vi "Configure Sweep.vi"(5 "Frequency Stop (5E+7 Hz)":dbl=50000000.0, 6 "Frequency Step (0)":i32, 7 "Frequency Start (5E+7 Hz)":dbl=50000000.0, 8 "error in (no error)":errorcluster, 9 "Time-gated Period (0.0001 s)":dbl=0.0001, 10 "Sweep Delay (0 s)":dbl, 11 "VISA resource name":refnum<visa-resource-name>) -> (0 "error out":errorcluster, 3 "VISA resource name out":refnum<visa-resource-name>)   [LabVIEW 2018, in "Agilent U2000 Series.lvlib"]
doc: "Changes the configurations for sweep mode.\n\nNote:\nThis VI is not applicable for Agilent U2021/2XA. In case of U2040 X-Series, it's applicable for U2042XA/U2044XA/U2049XA only."
uses:
  Agilent U2000 Series.lvlib
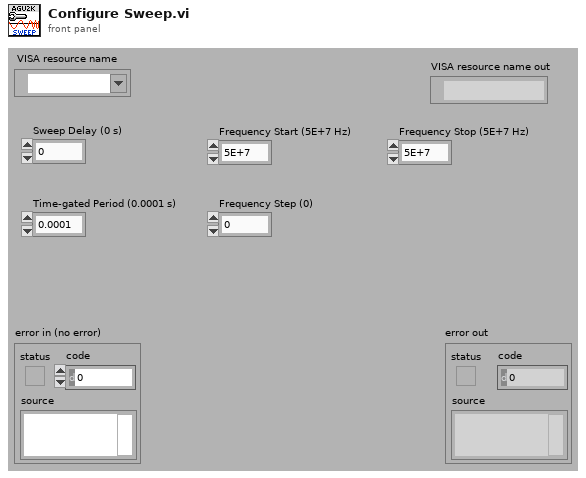
[diagram p1: front panel]
types:
  T1 = typedef "Agilent U2000 Series.lvlib/Extended User Data.ctl" = cluster{"U2000 Series Mode":u16, "Trigger Source Int/Ext":bool}
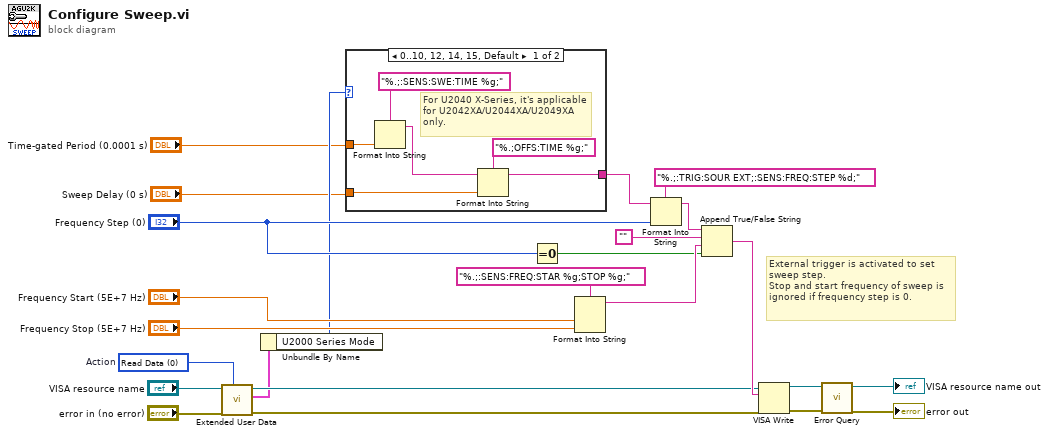
[diagram p0: block diagram]
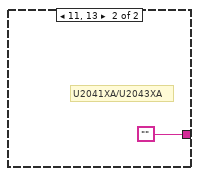
[diagram p2: hidden frame]
diagram:
  w1 = 0 items=["Read Data", "Write Data", "Clear Data", "Clear ALL Data"]  # Action
  # "External trigger is activated to set sweep step.\nStop and start frequency of sweep is ignored if frequency step is 0."
  n1 = call "Extended User Data.vi"("Action (1: Write Data)"=w1, "error in (no error)"="error in (no error)", "VISA resource name"="VISA resource name") -> ("error out"=w7:errorcluster, "User Data Out"=w6:T1, "VISA resource name out"=w8:refnum<visa-resource-name>)  [unwired: 6 in]
  n2 = Unbundle By Name(w6) -> ("U2000 Series Mode"=w5:u16)
  n3 = case shown="0..10, 12, 14, 15, Default" w5 {
    tunnel: "Time-gated Period (0.0001 s)" -> [w27 _]
    tunnel: "Sweep Delay (0 s)" -> [w26 _]
    tunnel: [w25 ""] -> w2
    frame 0..10, 12, 14, 15, Default {
      # "For U2040 X-Series, it's applicable for U2042XA/U2044XA/U2049XA only."
      n4 = Format Into String(format string="%.;:SENS:SWE:TIME %g;", w27) -> (resulting string=w28:string)  [unwired: 2 in, 1 out]
      n5 = Format Into String(format string="%.;OFFS:TIME %g;", initial string=w28, w26) -> (resulting string=w25:string)  [unwired: 1 in, 1 out]
    }
    frame 11, 13 {
      # "U2041XA/U2043XA"
    }
  }
  n6 = Equal To 0?(x="Frequency Step (0)") -> (x = 0?=w16:bool)
  n7 = Format Into String(format string="%.;:SENS:FREQ:STAR %g;STOP %g;", "Frequency Start (5E+7 Hz)", "Frequency Stop (5E+7 Hz)") -> (resulting string=w17:string)  [unwired: 2 in, 1 out]
  n8 = Format Into String(format string="%.;:TRIG:SOUR EXT;:SENS:FREQ:STEP %d;", initial string=w2, "Frequency Step (0)") -> (resulting string=w20:string)  [unwired: 1 in, 1 out]
  n9 = Append True/False String(1:w16, 2:w17, 3:"", 4:w20) -> (0:w11:string)
  n10 = VISA Write(VISA resource name=w8, write buffer=w11, error in (no error)=w7) -> (VISA resource name out=w24:refnum<visa-resource-name>, error out=w23:errorcluster)  [unwired: 1 out]
  n11 = call "Error Query.vi"("error in (no error)"=w23, "VISA resource name"=w24) -> ("error out"=→"error out":errorcluster, "VISA resource name out"=→"VISA resource name out":refnum<visa-resource-name>)  [unwired: 8 out]
